vi "QueryServer_Stop.vi"(0 "Server Info":T2, 2 "Event Registration Refnum":refnum<event-registration>, 3 "error in (no error)":errorcluster) -> (10 "error out":errorcluster)   [LabVIEW 2019, in "labview-grpc-query-server.lvlib"]
uses:
  labview-grpc-query-server.lvlib
  QueryServer_InvokeEventData.ctl
  QueryServer_gRPCid.ctl
  build/Debug/labview_grpc_server.dll
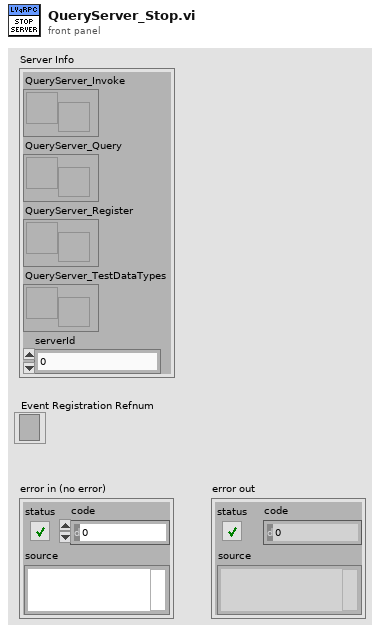
[diagram p1: front panel]
types:
  T1 = typedef "labview-grpc-query-server.lvlib/QueryServer_gRPCid.ctl" = u64
  T2 = cluster{"QueryServer_Invoke":refnum<user-event>, "QueryServer_Query":refnum<user-event>, "QueryServer_Register":refnum<user-event>, "QueryServer_TestDataTypes":refnum<user-event>, "serverId":T1}
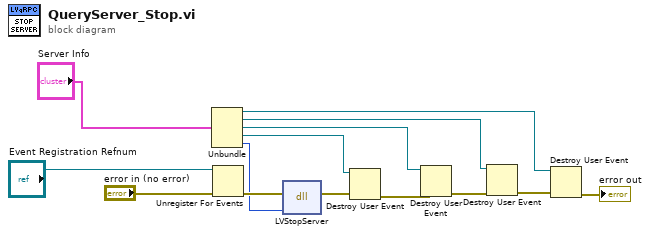
[diagram p0: block diagram]
diagram:
  n1 = Unbundle("Server Info") -> ("QueryServer_Invoke"=w7:refnum<user-event>, "QueryServer_Query"=w8:refnum<user-event>, "QueryServer_Register"=w9:refnum<user-event>, "QueryServer_TestDataTypes"=w1:refnum<user-event>, "serverId"=w4:T1)
  n2 = Unregister For Events(event registration refnum="Event Registration Refnum", error in="error in (no error)") -> (error out=w14:errorcluster)
  n3 = dll-call lib="C:/dev/labview-grpc-server/build/Debug/labview_grpc_server.dll" fn="LVStopServer"(error in=w14, "server"=w4) -> (error out=w3:errorcluster)  [unwired: 4 in, 1 out]
  n4 = Destroy User Event(user event=w1, error in=w3) -> (error out=w2:errorcluster)
  n5 = Destroy User Event(user event=w9, error in=w2) -> (error out=w12:errorcluster)
  n6 = Destroy User Event(user event=w8, error in=w12) -> (error out=w11:errorcluster)
  n7 = Destroy User Event(user event=w7, error in=w11) -> (error out=→"error out":errorcluster)
